vi "Set View Window Title.vi"(8 "error in (no error)":errorcluster, 11 "View In":refnum<class "View.lvclass">) -> (0 "error out":errorcluster, 3 "View Out":refnum<class "View.lvclass">)   [LabVIEW 2020, in "View.lvclass"]
uses:
  View.lvclass
  C:/git/astemes-triarc-framework/source/Framework/Process/Process.lvclass
  Process/Process.lvclass
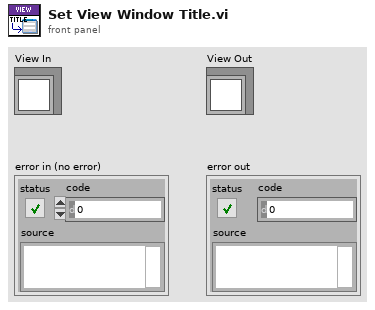
[diagram p1: front panel]
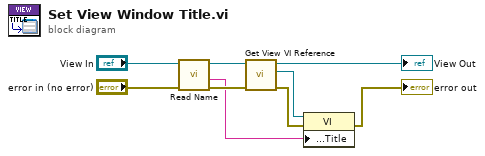
[diagram p0: block diagram]
diagram:
  n1 = call "Read Name.vi"("error in (no error)"="error in (no error)", "Process In"="View In") -> ("error out"=w8:errorcluster, "Name"=w7:string, "Process Out"=w3:refnum<class "View.lvclass">)  [unwired: 6 in, 1 out]
  n2 = call "Get View VI Reference.vi"("error in (no error)"=w8, "View In"=w3) -> ("error out"=w4:errorcluster, "View VI Reference"=w1:refnum<vi>, "View Out"=→"View Out":refnum<class "View.lvclass">)  [unwired: 7 in]
  n3 = property class="VI"(reference=w1, error in=w4, "Front Panel.Title"=w7) -> (error out=→"error out":errorcluster)  [unwired: 1 out]
